vi "Auto Arm Control.vi"(0 "Upper Arm Rollers":dbl, 1 "Upper Arms Open":bool, 3 "Upper Arms Close":bool, 9 "Lower Roller Left":dbl, 11 "Lower Roller Right":dbl, 12 "Lower Arm Extend":bool, 14 "Lower Arm Retract":bool) -> ()   [LabVIEW 2014]
uses:
  <vilib>/Rock Robotics/WPI/Solenoid/Deprecated/WPI_SolenoidSetBool.vi
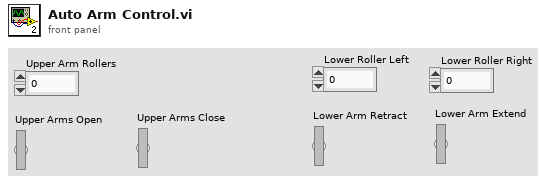
[diagram p1: front panel]
types:
  T1 = typedef "WPI_SolenoidDevRef.ctl" = cluster{"DevStatus":errorcluster, "Pneumatics Control Module":u8, "Forward Solenoid Channel":T2, "Reverse Solenoid Channel":T2}
  T2 = typedef "WPI_SolenoidChannel.ctl" = enum8{"Solenoid 0", "Solenoid 1", "Solenoid 2", "Solenoid 3", "Solenoid 4", "Solenoid 5", "Solenoid 6", "Solenoid 7", "Invalid"}
  T3 = typedef "WPI_MotorControlDeviceRef.ctl" = cluster{"DeviceStatus":errorcluster, "Type":T4, "PWM":cluster{"Controller":T5, "PWM Channel":T6, "DeadBand":T7}, "CAN":cluster{"Device Number":u8, "Control Mode":T8, "Semaphore":T9, "Max Vout":dbl, "TalonSRX Control Mode":T10}, "Invert":bool, "TransformRef":T11, "InvTransformRef":T11}
  T4 = typedef "WPI_MotorControlType.ctl" = enum16{"PWM", "CAN", "CANTalonSRX"}
  T5 = typedef "FPGA_TypedefDigitalModule.ctl" = enum16{"Controller 1"}
  T6 = typedef "FPGA_DIOPWMChannel.ctl" = enum8{"PWM 0", "PWM 1", "PWM 2", "PWM 3", "PWM 4", "PWM 5", "PWM 6", "PWM 7", "PWM 8", "PWM 9", "PWM MXP 0", "PWM MXP 1", "PWM MXP 2", "PWM MXP 3", "PWM MXP 4", "PWM MXP 5", "PWM MXP 6", "PWM MXP 7", "PWM MXP 8", "PWM MXP 9", "Invalid"}
  T7 = typedef "WPI_PWMDeadband.ctl" = cluster{"Name":string, "maxPositivePwm":i32, "minPositivePwm":i32, "centerPwm":i32, "maxNegativePwm":i32, "minNegativePwm":i32, "angularRange":u16}
  T8 = typedef "WPI_CANJaguar_ControlMode.ctl" = enum8{"Percent VBus", "Current", "Speed", "Position", "Voltage"}
  T9 = typedef "Semaphore RefNum" = refnum<k1>
  T10 = typedef "WPI_CANTalonSRX_APIControlMode.ctl" = enum8{"Percent VBus", "Speed", "Position", "Slave", "Unchanged / Invalid"}
  T11 = typedef "WPI_PWMTransform_ConPane.ctl" = refnum<vi>
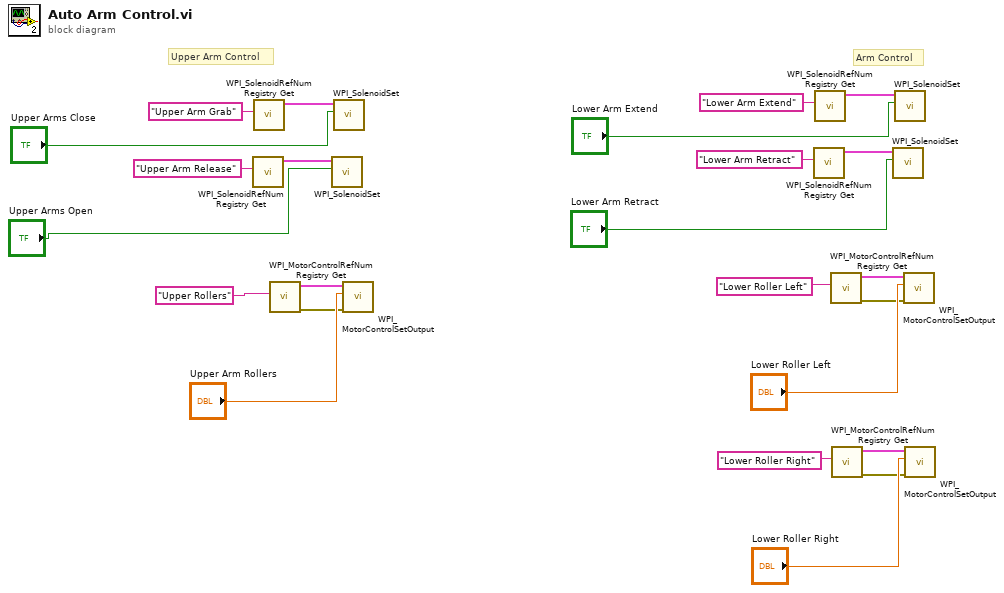
[diagram p0: block diagram]
diagram:
  # "Arm Control"
  # "Upper Arm Control"
  n1 = call <vilib>:"WPI_SolenoidRefNum Registry Get.vi"("refnum name"="Upper Arm Release") -> ("SolenoidDevRef"=w18:T1)  [unwired: 9 in, 1 out]
  n2 = call <vilib>:"WPI_SolenoidRefNum Registry Get.vi"("refnum name"="Upper Arm Grab") -> ("SolenoidDevRef"=w16:T1)  [unwired: 9 in, 1 out]
  n3 = call <vilib>:"WPI_MotorControlRefNum Registry Get.vi"("refnum name"="Upper Rollers") -> ("error out"=w22:errorcluster, "MotorControlDevRef"=w21:T3)  [unwired: 9 in]
  n4 = call-poly <vilib>:"WPI_SolenoidSet.vi"("Value"="Upper Arms Open", "SolenoidDevRef"=w18) -> ()  [unwired: 8 in, 2 out]
  n5 = call-poly <vilib>:"WPI_SolenoidSet.vi"("Value"="Upper Arms Close", "SolenoidDevRef"=w16) -> ()  [unwired: 8 in, 2 out]
  n6 = call <vilib>:"WPI_MotorControlSetOutput.vi"("error in (no error)"=w22, "Output"="Upper Arm Rollers", "MotorControlDevRef"=w21) -> ()  [unwired: 6 in, 3 out]
  n7 = call <vilib>:"WPI_SolenoidRefNum Registry Get.vi"("refnum name"="Lower Arm Retract") -> ("SolenoidDevRef"=w8:T1)  [unwired: 9 in, 1 out]
  n8 = call <vilib>:"WPI_SolenoidRefNum Registry Get.vi"("refnum name"="Lower Arm Extend") -> ("SolenoidDevRef"=w6:T1)  [unwired: 9 in, 1 out]
  n9 = call <vilib>:"WPI_MotorControlRefNum Registry Get.vi"("refnum name"="Lower Roller Left") -> ("error out"=w12:errorcluster, "MotorControlDevRef"=w11:T3)  [unwired: 9 in]
  n10 = call <vilib>:"WPI_MotorControlRefNum Registry Get.vi"("refnum name"="Lower Roller Right") -> ("error out"=w2:errorcluster, "MotorControlDevRef"=w1:T3)  [unwired: 9 in]
  n11 = call-poly <vilib>:"WPI_SolenoidSet.vi"("Value"="Lower Arm Retract", "SolenoidDevRef"=w8) -> ()  [unwired: 8 in, 2 out]
  n12 = call-poly <vilib>:"WPI_SolenoidSet.vi"("Value"="Lower Arm Extend", "SolenoidDevRef"=w6) -> ()  [unwired: 8 in, 2 out]
  n13 = call <vilib>:"WPI_MotorControlSetOutput.vi"("error in (no error)"=w12, "Output"="Lower Roller Left", "MotorControlDevRef"=w11) -> ()  [unwired: 6 in, 3 out]
  n14 = call <vilib>:"WPI_MotorControlSetOutput.vi"("error in (no error)"=w2, "Output"="Lower Roller Right", "MotorControlDevRef"=w1) -> ()  [unwired: 6 in, 3 out]
